vi "peak-poly-fit .vi"() -> ()   [LabVIEW 2013]
uses:
  <vilib>/Analysis/NI_AALPro.lvlib
panel:
  out "Max_x":dbl
  out "a":dbl
  out "fit data":cluster{"Best Polynomial Fit":dbl[], dbl[]}
  in  "array_y":dbl[](array[numeric])
  in  "array_x":dbl[](array[numeric])
  in  "half length":i32=1
  out "out-of-range":bool
  in  "error in (no error)":errorcluster caption="错误输入（无错误）"
  out "error out":errorcluster caption="错误输出"
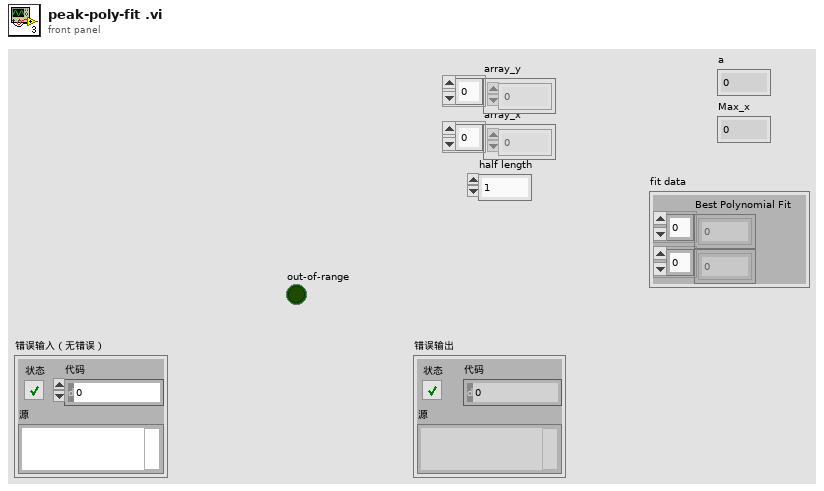
[diagram p1: front panel]
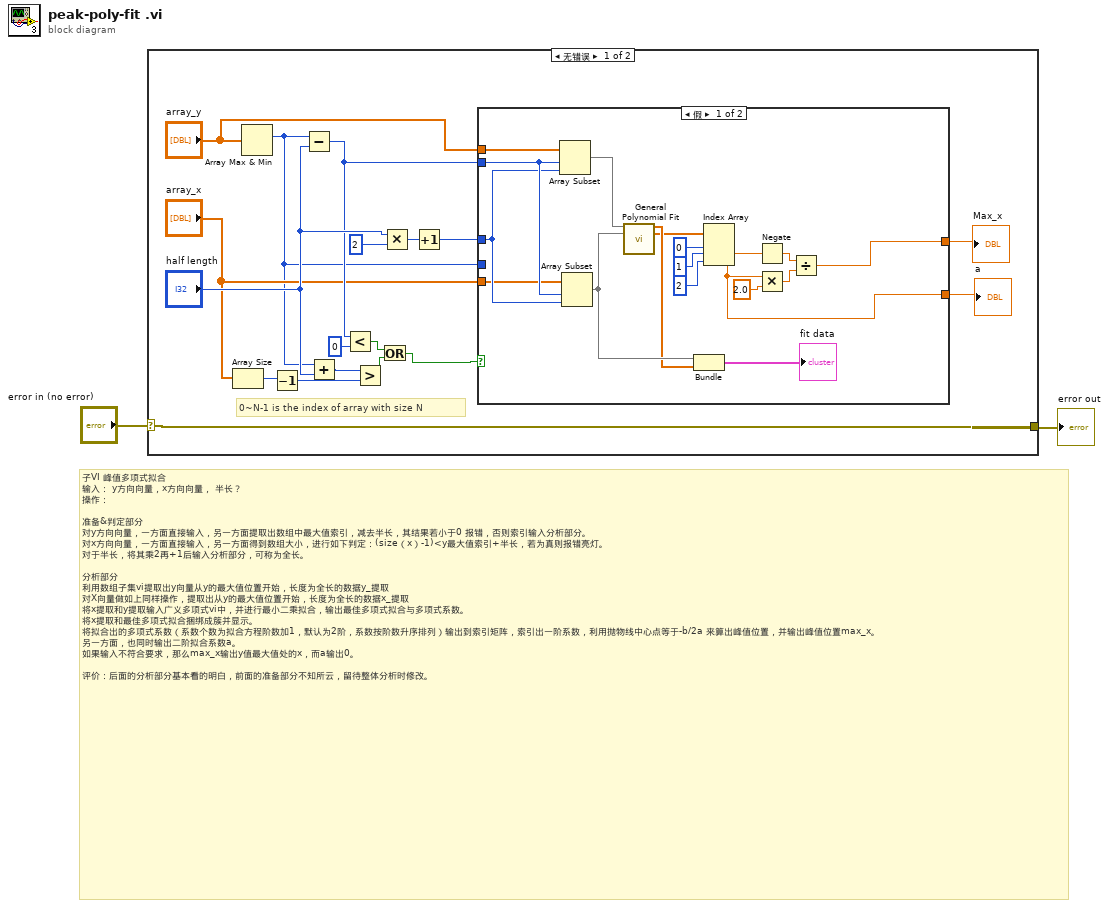
[diagram p0: block diagram]
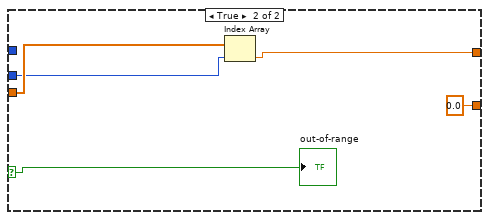
[diagram p2: hidden frame]
diagram:
  # "子VI 峰值多项式拟合\n输入： y方向向量，x方向向量， 半长？\n操作：\n\n准备&判定部分\n对y方向向量，一方面直接输入，另一方面提取出数组中最大值索引，减去半长，其结果若小于0 报错，否则索引输入分析部分。\n对x方向向量，一方面直接输入，另一方面得到数组大小，进行如下判定：(size（x）-1)<y最大值索引+半长，若为真则报错亮灯。\n对于半长，将其乘2再+1后输入分析部分，可称为全长。\n\n分析部分\n利用数组子集vi提取出y向量从y的最大值位置开始，长度为全长的数据y_提取\n对X向量做如上同样操作，提取出从y的最大值位置开始，长度为全长的数据x_提取\n将x提取和y提取输入广义多项式vi中，并进行最小二乘拟合，输出最佳多项式拟合与多项式系数。\n将x提取和最佳多项式拟合捆绑成簇并显示。\n将拟合出的多项式系数（系数个数为拟合方程阶数加1，默认为2阶，系数按阶数升序排列）输出到索引矩阵，索引出一阶系数，利用抛物线中心点等于-b/2a 来算出峰值位置，并输出峰值位置max_x。\n另一方面，也同时输出二阶拟合系数a。\n如果输入不符合要求，那么max_x输出y值最大值处的x，而a输出0。\n\n评价：后面的分析部分基本看的明白，前面的准备部分不知所云，留待整体分析时修改。"
  n1 = case shown="无错误" "error in (no error)" {
    selector: "error in (no error)" -> [w20 w44]
    tunnel: [w20 w44] -> w2
    frame No Error {
      # "0~N-1 is the index of array with size N"
      n2 = Array Size(array="array_x") -> (size(s)=w18:i32)
      n3 = Array Max & Min(array="array_y") -> (max index (indices)=w3:i32)  [unwired: 3 out]
      n4 = Decrement(x=w18) -> (x-1=w17:i32)
      n5 = Subtract(x=w3, y="half length") -> (x-y=w8:i32)
      n6 = Add(x=w3, y="half length") -> (x+y=w14:i32)
      n7 = Less?(x=w8, y=0) -> (x < y?=w15:bool)
      n8 = Greater?(x=w14, y=w17) -> (0:w16:bool)
      n9 = Or(x=w15, y=w16) -> (x .or. y?=w10:bool)
      n10 = Multiply(x="half length", y=2) -> (x*y=w11:i32)
      n11 = Increment(x=w11) -> (x+1=w7:i32)
      n12 = case shown="假" w10 {
        selector: w10 -> [_ w43]
        tunnel: "array_y" -> [w26 _]
        tunnel: w8 -> [w25 _]
        tunnel: w7 -> [w24 _]
        tunnel: "array_x" -> [w23 w42]
        tunnel: [w22 w40] -> w5
        tunnel: [w21 0.0] -> w4
        tunnel: w3 -> [_ w41]
        frame False {
          n13 = Array Subset(array=w26, index=w25, length=w24) -> (w27:dbl[])
          n14 = Array Subset(array=w23, index=w25, length=w24) -> (w38:dbl[])
          n15 = call <vilib>:"General Polynomial Fit.vi"("Y"=w27, "X"=w38) -> ("Best Polynomial Fit"=w37:dbl[], "Polynomial Coefficients"=w28:dbl[])  [unwired: 10 in, 2 out]
          n16 = Bundle(w38, "Best Polynomial Fit"=w37) -> (→"fit data":cluster{dbl[], "Best Polynomial Fit":dbl[]})  [unwired: 1 out]
          n17 = Index Array(array=w28, index #1=0 ("index"), index #2=1 ("index"), index #3=2 ("index")) -> (element #2=w32:dbl, element #3=w21:dbl)  [unwired: 1 out]
          n18 = Negate(x=w32) -> (-x=w35:dbl)
          n19 = Multiply(x=w21, y=2.0) -> (x*y=w34:dbl)
          n20 = Divide(x=w35, y=w34) -> (x/y=w22:dbl)
        }
        frame True {
          n21 = Index Array(array=w42, index=w41) -> (element=w40:dbl)
          "out-of-range" <- w43
        }
      }
      "Max_x" <- w5
      "a" <- w4
    }
    frame Error {
    }
  }
  "error out" <- w2
